vi "KeyDown.vi"(1 "Virtual Key":u8(ring)=65) -> ()   [LabVIEW 2015]
uses:
  user32.dll
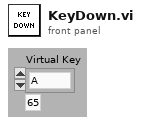
[diagram p1: front panel]
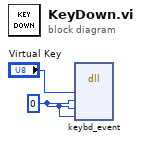
[diagram p0: block diagram]
diagram:
  w2 = u8 0 ("bScan")
  n1 = dll-call lib="user32.dll" fn="keybd_event" label="user32.dll void  keybd_event(uint8_t bVk, uint8_t bScan, uint32_t dwFlags, uint32_t dwExtraInfo);"("bVk"="Virtual Key", "bScan"=w2, "dwFlags"=w2, "dwExtraInfo"=w2) -> ()  [unwired: 8 in, 2 out]
